vi "Linear Filter.vi"(4 "Error":string, 5 "Mask":i8[][](array[numeric]), 6 "Output Image":T1={"Image ID"=0, "Channel ID"=-1}, 7 "Input Image":T1={"Image ID"=0, "Channel ID"=-1}) -> (0 "Error":string, 2 "Output Image":T1={"Image ID"=0, "Channel ID"=-1}, 3 "Input Image":T1={"Image ID"=0, "Channel ID"=-1})   [LabVIEW 2011, in "labvvis.lvlib"]
doc: "Divides the sum of the multiplication of the pixels from Input Image with the Mask, by the sum of the values in the Mask.\n\nExamples of Linear Filters are gradient filters, Laplacian filters, smoothing filters and Gaussian filters."
uses:
  <userlib>/labvvis/labvvis.lvlib
  <userlib>/labvvis/VVIS Image.ctl
  labvvis.framework
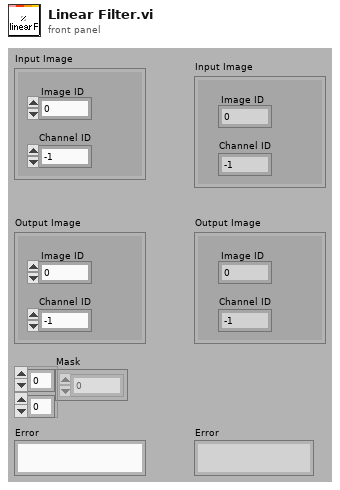
[diagram p1: front panel]
types:
  T1 = typedef "labvvis.lvlib/VVIS Image.ctl" = cluster{"Image ID":i16, "Channel ID":i16}
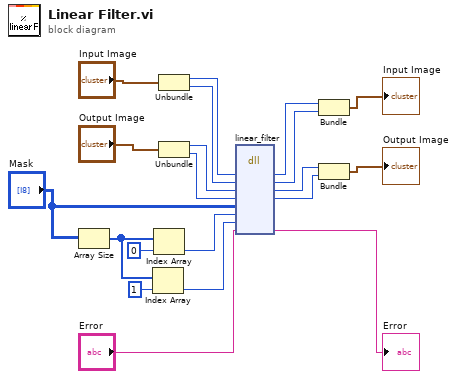
[diagram p0: block diagram]
diagram:
  n1 = Array Size(array="Mask") -> (size(s)=w17:i32[])
  n2 = Index Array(array=w17, index=1) -> (element=w5:i32)
  n3 = Index Array(array=w17, index=0) -> (element=w6:i32)
  n4 = Unbundle("Input Image") -> ("Image ID"=w15:i16, "Channel ID"=w12:i16)
  n5 = Unbundle("Output Image") -> ("Image ID"=w11:i16, "Channel ID"=w10:i16)
  n6 = dll-call lib="labvvis.framework" fn="linear_filter"("src1"=w15, "icid"=w12, "out"=w11, "ocid"=w10, "mask"="Mask", "kw"=w6, "kh"=w5, "error"="Error") -> ("src1"=w14:i16, "icid"=w9:i16, "out"=w8:i16, "ocid"=w7:i16, "error"=→"Error":string)  [unwired: 7 in, 2 out]
  n7 = Bundle("src1"=w14, "icid"=w9) -> (→"Input Image":cluster{"src1":i16, "icid":i16})  [unwired: 1 in]
  n8 = Bundle("out"=w8, "ocid"=w7) -> (→"Output Image":cluster{"out":i16, "ocid":i16})  [unwired: 1 in]
